vi "setup_fpga_daq (SubVI).vi"(9 "config_trig":dbl[](array[numeric]) format="%0.2f", 10 "file_path_cluster":T2, 11 "channel_settings":T1) -> ()   [LabVIEW 2018]
uses:
  <vilib>/DAQmx/write.llb/DAQmx Write (Analog 1D DBL 1Chan NSamp).vi
  <vilib>/DAQmx/create/channels.llb/DAQmx Create Channel (AO-Voltage-Basic).vi
  <vilib>/DAQmx/configure/timing.llb/DAQmx Timing (Sample Clock).vi
  <vilib>/DAQmx/miscellaneous.llb/DAQmx Fill In Error Info.vi
  <vilib>/DAQmx/configure/trigger.llb/DAQmx Start Trigger (None).vi
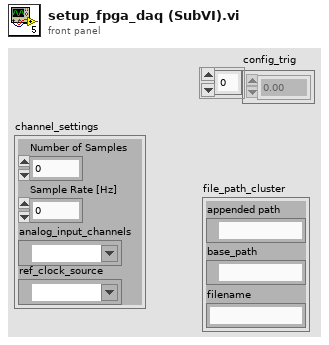
[diagram p1: front panel]
types:
  T1 = cluster{"Number of Samples":i32, "Sample Rate [Hz]":dbl, "analog_input_channels":tag, "ref_clock_source":tag}
  T2 = cluster{"appended path":path, "base_path":path, "filename":string}
  T3 = enum16{"open", "replace", "create", "open or create", "replace or create", "replace or create with confirmation"}
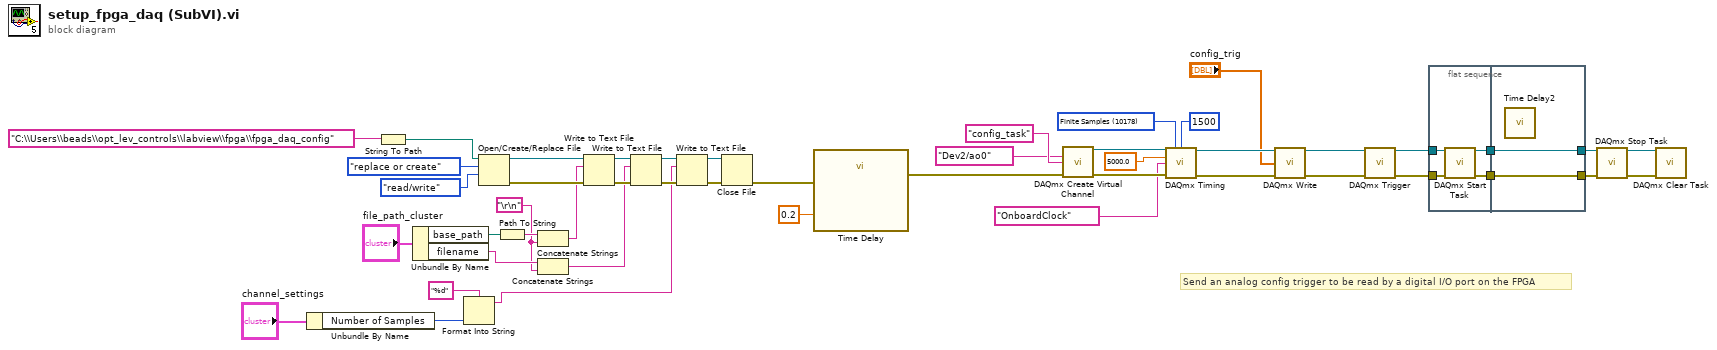
[diagram p0: block diagram]
diagram:
  w24 = "\r\n" ("format string")
  w43 = 10178 items=["Finite Samples"=10178, "Continuous Samples"=10123, "Hardware Timed Single Point"=12522] ("sample mode")
  # "Send an analog config trigger to be read by a digital I/O port on the FPGA"
  n1 = Unbundle By Name("channel_settings") -> ("Number of Samples"=w18:i32)
  n2 = String To Path(string="C:\\Users\\beads\\opt_lev_controls\\labview\\fpga\\fpga_daq_config") -> (path=w32:path)
  n3 = Unbundle By Name("file_path_cluster") -> ("base_path"=w39:path, "filename"=w25:string)
  n4 = Format Into String(format string="%d", w18) -> (resulting string=w20:string)  [unwired: 2 in, 1 out]
  n5 = Open/Create/Replace File(file path (use dialog)=w32, operation (0:open)=T3."replace or create", access (0:read/write)=enum16{"read/write", "read-only", "write-only"}."read/write") -> (refnum out=w36:refnum<file>, error out=w35:errorcluster)  [unwired: 3 in, 1 out]
  n6 = Path To String(path=w39) -> (string=w31:string)
  n7 = Concatenate Strings(w31, w24) -> (w30:string)
  n8 = Concatenate Strings(w25, w24) -> (w23:string)
  n9 = Write to Text File(file (use dialog)=w36, text=w30, error in=w35) -> (refnum out=w29:refnum<file>, error out=w28:errorcluster)  [unwired: 1 in, 1 out]
  n10 = Write to Text File(file (use dialog)=w29, text=w23, error in=w28) -> (refnum out=w27:refnum<file>, error out=w26:errorcluster)  [unwired: 1 in, 1 out]
  n11 = Write to Text File(file (use dialog)=w27, text=w20, error in=w26) -> (refnum out=w22:refnum<file>, error out=w21:errorcluster)  [unwired: 1 in, 1 out]
  n12 = Close File(refnum=w22, error in=w21) -> (error out=w19:errorcluster)  [unwired: 1 out]
  n13 = call "Time Delay"("error in (no error)"=w19, "Delay Time (s)"=0.2) -> ("error out"=w42:errorcluster)  [unwired: 9 in]
  n14 = call-poly <vilib>:"DAQmx Create Virtual Channel.vi"("physical channels"=tag "Dev2/ao0", "name to assign"="config_task", "error in"=w42) -> ("task out"=w45:refnum<k21>, "error out"=w46:errorcluster)  [unwired: 11 in]
  n15 = call-poly <vilib>:"DAQmx Timing.vi"("task/channels in"=w45, "sample mode"=w43, "samples per channel"=1500, "rate"=5000.0, "source"=tag "OnboardClock", "error in"=w46) -> ("task out"=w10:refnum<k21>, "error out"=w9:errorcluster)  [unwired: 8 in]
  n16 = call-poly <vilib>:"DAQmx Write.vi"("task/channels in"=w10, "data"="config_trig", "error in"=w9) -> ("task out"=w5:refnum<k21>, "error out"=w4:errorcluster)  [unwired: 10 in, 1 out]
  n17 = call-poly <vilib>:"DAQmx Trigger.vi"("task/channels in"=w5, "error in"=w4) -> ("task out"=w2:refnum<k21>, "error out"=w3:errorcluster)  [unwired: 12 in]
  n18 = flat-sequence {
    tunnel: w2 -> [w49]
    tunnel: w3 -> [w48]
    tunnel: [w51] -> w8
    tunnel: [w50] -> w7
    tunnel: [w52] -> w13
    tunnel: [w53] -> w14
    tunnel: w8 -> [w53]
    tunnel: w7 -> [w52]
    frame #0 {
      n19 = call <vilib>:"DAQmx Start Task.vi"("task/channels in"=w49, "error in"=w48) -> ("task out"=w51:refnum<k21>, "error out"=w50:errorcluster)  [unwired: 12 in]
    }
    frame #1 {
      n20 = call "Time Delay2"() -> ()  [unwired: 11 in, 1 out]
    }
  }
  n21 = call <vilib>:"DAQmx Stop Task.vi"("task/channels in"=w14, "error in"=w13) -> ("task out"=w16:refnum<k21>, "error out"=w15:errorcluster)  [unwired: 12 in]
  n22 = call <vilib>:"DAQmx Clear Task.vi"("task in"=w16, "error in"=w15) -> ()  [unwired: 13 in, 1 out]
